vi "Set Selected Aircraft.vi"(8 "Error In":errorcluster, 11 "Selected Aircraft ID In":u8) -> (0 "Error Out":errorcluster)   [LabVIEW 2014]
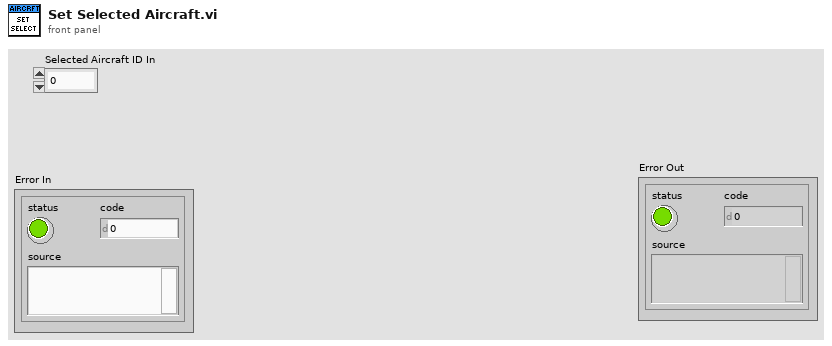
[diagram p1: front panel]
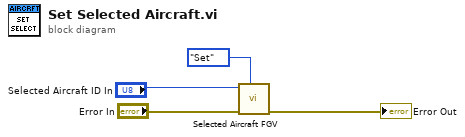
[diagram p0: block diagram]
diagram:
  n1 = call "Selected Aircraft FGV.vi"("Operation"=enum16{"Get", "Set"}."Set", "Error In"="Error In", "Selected Aircraft ID In"="Selected Aircraft ID In") -> ("Error Out"=→"Error Out":errorcluster)  [unwired: 7 in, 1 out]
